vi "Balance.vi"() -> ()   [LabVIEW 2014]
uses:
  <userlib>/UCSD Robotics Lab/Robotics-Cape/LV/libroboticscape.lvlib
panel:
  in  "Fast Loop Gain Multiplier":dbl=1.0
  out "State":T1(ring)
  in  "Slow Loop Gain Multiplier":dbl=1.0
  in  "Gamma Setpoint":dbl
  in  "Phi Setpoint":dbl step=0.25
  in  "Steering On/off":bool=TRUE
  out "Slow Loop State":T2 {"Phi Setpoint" format="%#_13g"; "Phi" format="%#_4g"; "error Phi" format="%#_4g"; "Gamma" format="%#_4g"}
  out "Actual Loop rate (Hz)":dbl format="%#_4g"
  out "Armed Status":bool
  out "Fast Loop State":T3 {"Theta (Deg)" format="%#_3g"; "Theta (Rad)" format="%#_3g"; "eTheta" format="%#_3g"; "Steering U" format="%#_2g"}
  in  "Controller - User Input":T4={"Num Fast Loop"=[-5.391, 10.21, -4.829], "Den Fast Loop"=[1.0, -1.702, 0.702], "Fast Loop Gain"=1.0, "IMU_sample_rate"=200, "Num Slow Loop"=[0.28, -0.5581, 0.2781], "Den Slow Loop"=[1.0, -1.86, 0.8605], "Slow Loop Gain"=1.0, "Slow Loop sample rate"=100.0} {"Slow Loop sample rate" min=4.0 max=200.0; "IMU_sample_rate" min=4 max=200}
  in  "Steering PID Gains":T5={"proportional"=0.1, "integral"=0.05, "derivative"=0.0}
  out "Slow Loop Gains":T6
  out "Commanded  Slow Loop Sample rate":dbl
  in  "Controller Select":T7(ring)=enum."User Defined" caption="Enum"
  out "Fast Loop Gains":T8
  in  "Display Slow Loop":bool
  in  "Display Fast Loop":bool
  out "U Plot":cluster{"U saturated":sgl, "U":dbl}(graph)
  out "Theta Ref":cluster{"Filtered x":dbl, "val out":sgl}(graph)
  out "Slower Loop (Hz)":dbl format="%#_4g"
  out "Theta Plot":dbl(graph)
  out "IMU_sample_rate":i32=200
  in  "stop":bool
  # "Always stop the VI using the rectangular STOP button below, never with the round stopsign (Abort)"
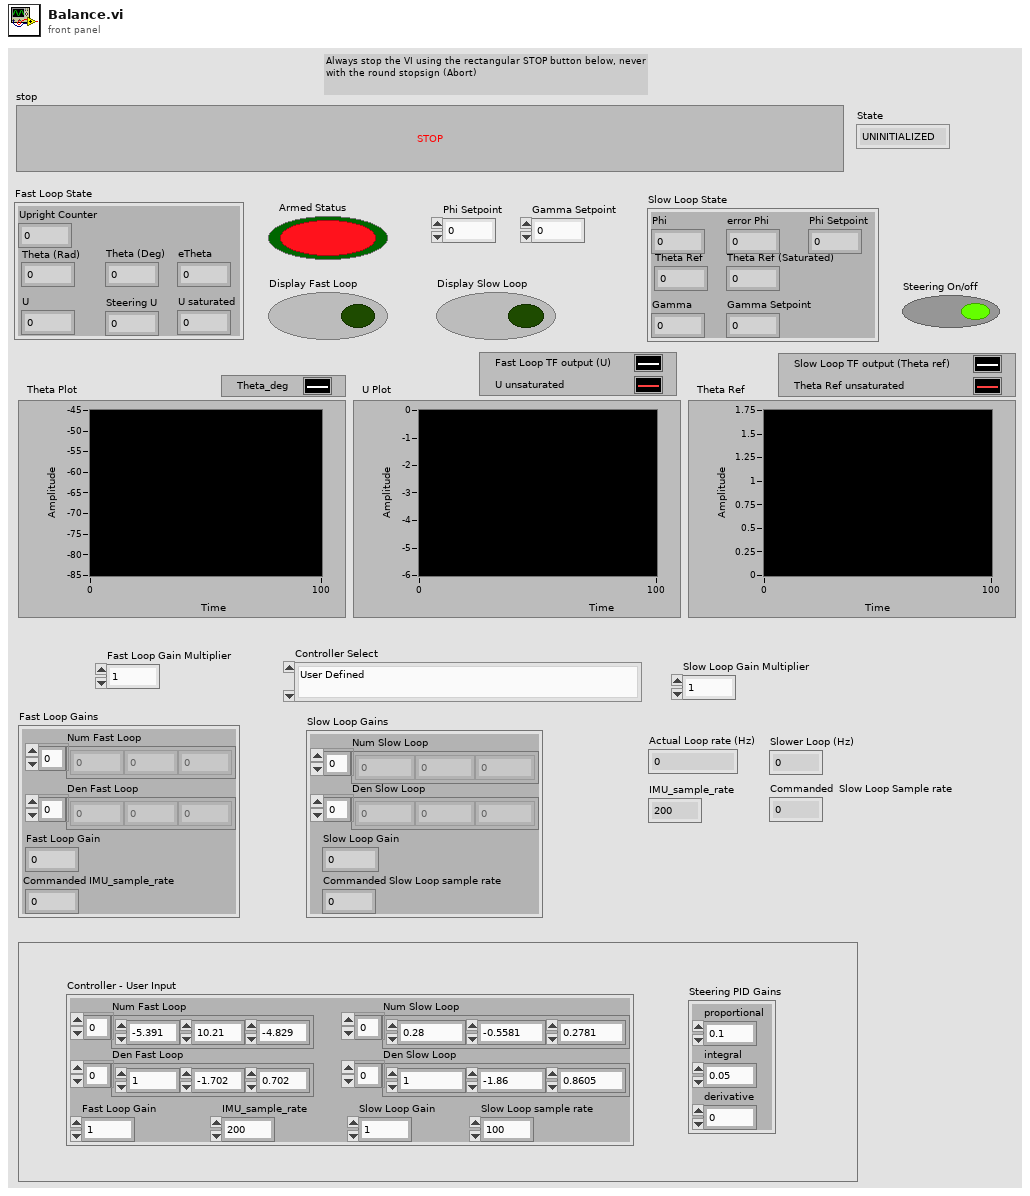
[diagram p1: front panel]
types:
  T1 = enum16{"UNINITIALIZED", "RUNNING", "PAUSED", "EXITING"}
  T2 = cluster{"Phi":dbl, "error Phi":dbl, "Gamma":dbl, "Theta Ref":dbl, "Theta Ref (Saturated)":sgl, "Gamma Setpoint":dbl, "Phi Setpoint":dbl}
  T3 = cluster{"Upright Counter":dbl, "Theta (Deg)":dbl, "Theta (Rad)":dbl, "eTheta":dbl, "U":dbl, "Steering U":dbl, "U saturated":sgl}
  T4 = cluster{"Num Fast Loop":dbl[], "Den Fast Loop":dbl[], "Fast Loop Gain":dbl, "IMU_sample_rate":i32, "Num Slow Loop":dbl[], "Den Slow Loop":dbl[], "Slow Loop Gain":dbl, "Slow Loop sample rate":dbl}
  T5 = cluster{"proportional":dbl, "integral":dbl, "derivative":dbl}
  T6 = cluster{"Num Slow Loop":dbl[], "Den Slow Loop":dbl[], "Slow Loop Gain":dbl, "Commanded Slow Loop sample rate":dbl}
  T7 = enum16{"100hz/50hz", "100hz/100hz", "200hz/200hz", "200hz/20hz", "User Defined"}
  T8 = cluster{"Num Fast Loop":dbl[], "Den Fast Loop":dbl[], "Fast Loop Gain":dbl, "Commanded IMU_sample_rate":i32}
  T9 = cluster{"accel[0]":sgl, "accel[1]":sgl, "accel[2]":sgl, "gyro[0]":sgl, "gyro[1]":sgl, "gyro[2]":sgl, "mag[0]":sgl, "mag[1]":sgl, "mag[2]":sgl, "temp":sgl, "raw_gyro[0]":i16, "raw_gyro[1]":i16, "raw_gyro[2]":i16, "raw_accel[0]":i16, "raw_accel[1]":i16, "raw_accel[2]":i16, "accel_to_ms2":sgl, "gyro_to_degs":sgl, "dmp_quat[0]":sgl, "dmp_quat[1]":sgl, "dmp_quat[2]":sgl, "dmp_quat[3]":sgl, "dmp_TaitBryan[0]":sgl, "dmp_TaitBryan[1]":sgl, "dmp_TaitBryan[2]":sgl, "fused_quat[0]":sgl, "fused_quat[1]":sgl, "fused_quat[2]":sgl, "fused_quat[3]":sgl, "fused_TaitBryan[0]":sgl, "fused_TaitBryan[1]":sgl, "fused_TaitBryan[2]":sgl, "compass_heading":sgl, "compass_heading_raw":sgl}
  T10 = enum16{"UNINITIALIZED", "RUNING", "PAUSED", "EXITING"}
  T11 = cluster{"Num Fast Loop":dbl[], "Den Fast Loop":dbl[], "Fast Loop Gain 3":dbl, "IMU_sample_rate":i32}
  T12 = cluster{"Upright Counter":dbl, "Theta (Deg)":dbl, "Theta (Rad)":dbl, "eTheta":dbl, "U":dbl, "Steering output":dbl, "U saturated":sgl}
  T13 = cluster{"Num Slow Loop":dbl[], "Den Slow Loop":dbl[], "Slow Loop Gain":dbl, "Commanded Slow Sample rate":dbl}
  T14 = cluster{"Theta Ref":dbl, "Theta Ref (Saturated)":sgl}
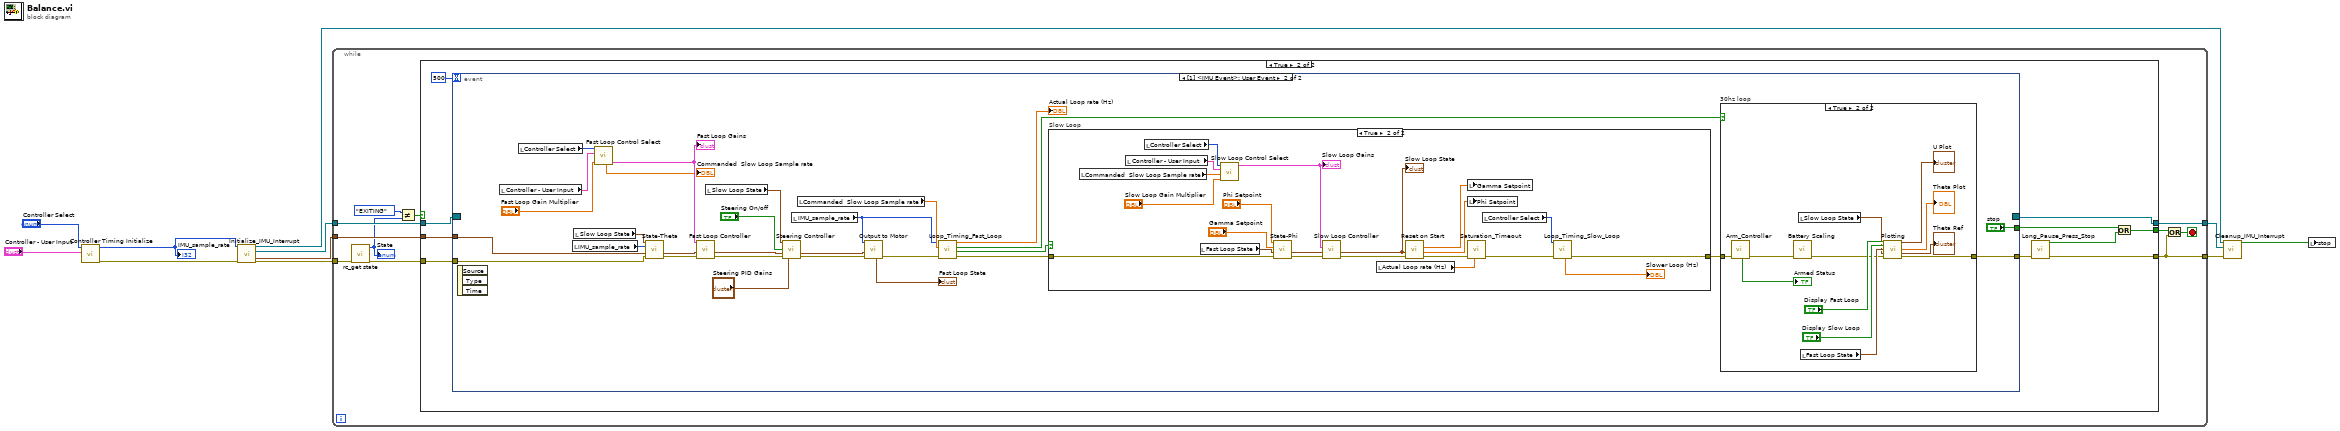
[diagram p0: block diagram]
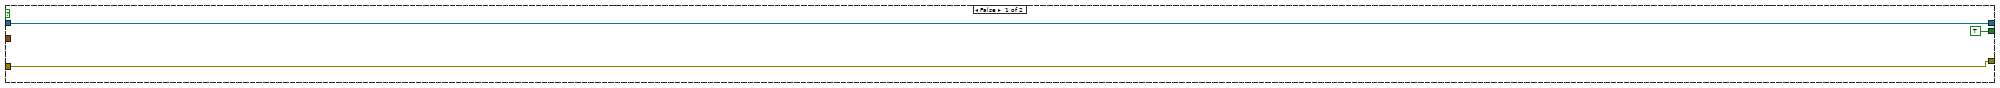
[diagram p2: hidden frame]
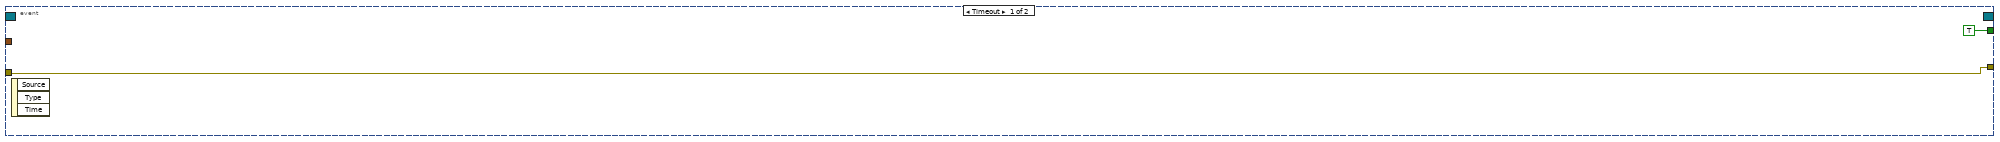
[diagram p3: hidden frame]
diagram:
  n1 = call "Controller Timing Initialize.vi"("Controller - User Input"="Controller - User Input", "Controller Select"="Controller Select") -> ("error out"=w2:errorcluster, "IMU_sample_rate"=w5:i32)  [unwired: 8 in]
  "IMU_sample_rate" <- w5
  n2 = call "Initialize_IMU_Interrupt.vi"("dmp_sample_rate"=w5, "error in (no error)"=w2) -> ("IMU Event"=w8:refnum<user-event>, "Event Registration Refnum"=w10:refnum<event-registration>, "IMU Data"=w6:T9, "error out"=w3:errorcluster)  [unwired: 10 in]
  n3 = while {
    tunnel: w3 -> [w17]
    tunnel: [w22] -> w7
    tunnel: [w20] -> w11
    tunnel: w10 -> [w21]
    tunnel: w6 -> [w18]
    stop <- w19 stop-if-true
    n4 = call <userlib>:"rc_get state.vi"("error in (no error)"=w17) -> ("error out"=w16:errorcluster, "function return"=w12:u32)  [unwired: 9 in]
    "State" <- w12
    n5 = Not Equal?(x=T10."EXITING" ("State 2"), y=w12) -> (x != y?=w14:bool)
    n6 = case shown="True" w14 {
      tunnel: [w24 w35] -> w22
      tunnel: w21 -> [w24 w33]
      tunnel: [w25 w29] -> w20
      tunnel: w18 -> [_ w32]
      tunnel: w16 -> [w25 w31]
      tunnel: [TRUE ("stop") w26] -> w13
      frame False {
      }
      frame True {
        n7 = event shown="[1] <IMU Event>: User Event" {
          selector: w33 -> [_ _]
          dyn-events: [_ _] -> w35
          timeout: 500 -> [_ _]
          tunnel: w31 -> [w37 w66]
          tunnel: [w37 w56] -> w30
          tunnel: w32 -> [_ w55]
          tunnel: [TRUE ("stop") "stop"] -> w27
          event Timeout {
            n8 = event-data() -> ()  [unwired: 1 in, 3 out]
          }
          event User Event {
            n9 = event-data() -> ()  [unwired: 1 in, 3 out]
            n10 = local read "Controller - User Input"() -> (w39:T4)
            n11 = local read "Controller Select"() -> (w43:T7)
            n12 = local read "IMU_sample_rate"() -> (w42:i32)
            n13 = local read "Slow Loop State"() -> (w45:T2)
            n14 = call "Fast Loop Control Select.vi"("Fast Loop Gain Multiplier"="Fast Loop Gain Multiplier", "Controller - User Input"=w39, "Controller Select"=w43) -> ("Fast Loop Controller"=w48:T11, "Slow Loop sample rate out"=→"Commanded  Slow Loop Sample rate":dbl)  [unwired: 7 in]
            "Fast Loop Gains" <- w48
            n15 = call "State-Theta.vi"("Slow Loop State in"=w45, "IMU_sample_rate"=w42, "IMU Data Struct in"=w55, "error in"=w66) -> ("Fast Loop State out"=w54:T12, "error out"=w65:errorcluster)  [unwired: 10 in]
            n16 = call "Fast Loop Controller.vi"("error in"=w65, "Fast Loop State in"=w54, "Fast Loop Controller in"=w48) -> ("error out"=w62:errorcluster, "Fast Loop State out"=w53:T12)  [unwired: 7 in]
            n17 = local read "Slow Loop State"() -> (w46:T2)
            n18 = call "Steering Controller.vi"("Slow Loop State in"=w46, "Steering On/off"="Steering On/off", "Fast Loop State in"=w53, "error in"=w62, "PID Gains in"="Steering PID Gains") -> ("Fast Loop State out"=w52:T12, "error out"=w61:errorcluster)  [unwired: 9 in]
            n19 = local read "IMU_sample_rate"() -> (w41:i32)
            n20 = local read "Commanded  Slow Loop Sample rate"() -> (w50:dbl)
            n21 = call "Output to Motor.vi"("error in (no error)"=w61, "Fast Loop State in"=w52, "IMU_sample_rate"=w41) -> ("error out"=w64:errorcluster, "Fast Loop State out"=→"Fast Loop State":T12)  [unwired: 7 in]
            n22 = call "Loop_Timing_Fast_Loop.vi"("error in"=w64, "Slow Loop sample rate in"=w50, "IMU_sample_rate in"=w41) -> ("error out"=w58:errorcluster, "Slow Loop Start"=w63:bool, "30hz Start"=w60:bool, "Hz"=→"Actual Loop rate (Hz)":dbl)  [unwired: 5 in]
            n23 = case "Slow Loop" shown="True" w63 {
              tunnel: [w80 w101] -> w57
              tunnel: w58 -> [w80 w96]
              frame False {
              }
              frame True {
                n24 = local read "Commanded  Slow Loop Sample rate"() -> (w99:dbl)
                n25 = local read "Controller - User Input"() -> (w98:T4)
                n26 = local read "Controller Select"() -> (w81:T7)
                n27 = local read "Fast Loop State"() -> (w97:T3)
                n28 = call "Slow Loop Control Select.vi"("Slow Loop Gain Multiplier"="Slow Loop Gain Multiplier", "Commanded Slow Sample rate"=w99, "Controller - User Input"=w98, "Controller Select"=w81) -> ("Slow Loop Gains"=w86:T13)  [unwired: 7 in]
                "Slow Loop Gains" <- w86
                n29 = call "State-Phi.vi"("error in (no error)"=w96, "Fast Loop State in"=w97, "Gamma Setpoint"="Gamma Setpoint", "Phi Setpoint"="Phi Setpoint") -> ("error out"=w100:errorcluster, "Slow Loop State out"=w85:T2)  [unwired: 6 in]
                n30 = call "Slow Loop Controller.vi"("error in"=w100, "Slow Loop State in"=w85, "Slow Loop Gains"=w86) -> ("error out"=w94:errorcluster, "Slow Loop State out"=w87:T2)  [unwired: 5 in]
                "Slow Loop State" <- w87
                n31 = local read "Actual Loop rate (Hz)"() -> (w95:dbl)
                n32 = call "Reset on Start.vi"("error in (no error)"=w94, "Slow Loop State"=w87) -> ("error out"=w93:errorcluster, "Phi Setpoint"=w89:dbl, "Gamma Setpoint"=w90:dbl)  [unwired: 6 in, 1 out]
                n33 = local write "Gamma Setpoint"(w90) -> ()
                n34 = local write "Phi Setpoint"(w89) -> ()
                n35 = call "Saturation_Timeout.vi"("Hz"=w95, "error in"=w93) -> ("error out"=w92:errorcluster)  [unwired: 9 in]
                n36 = local read "Controller Select"() -> (w82:T7)
                n37 = call "Loop_Timing_Slow_Loop.vi"("error in"=w92, "Controller Select"=w82) -> ("error out"=w101:errorcluster, "Hz"=→"Slower Loop (Hz)":dbl)  [unwired: 6 in, 2 out]
              }
            }
            n38 = case "30hz loop" shown="True" w60 {
              tunnel: w57 -> [w67 w79]
              tunnel: [w67 w78] -> w56
              frame False {
              }
              frame True {
                n39 = call "Arm_Controller.vi"("error in (no error)"=w79) -> ("error out"=w70:errorcluster, "Arm Controller"=→"Armed Status":bool)  [unwired: 8 in, 1 out]
                n40 = call "Battery Scaling.vi"("error in (no error)"=w70) -> ("error out"=w69:errorcluster)  [unwired: 9 in, 1 out]
                n41 = local read "Slow Loop State"() -> (w68:T2)
                n42 = local read "Fast Loop State"() -> (w75:T3)
                n43 = call "Plotting.vi"("Display Fast Loop"="Display Fast Loop", "Display Slow Loop"="Display Slow Loop", "Fast Loop State in"=w75, "Slow Loop State in"=w68, "error in (no error)"=w69) -> ("U plot"=→"U Plot":cluster{"U saturated":sgl, "U":dbl}, "Theta (Deg)"=→"Theta Plot":dbl, "Theta Ref Plot"=→"Theta Ref":T14, "error out"=w78:errorcluster)  [unwired: 7 in]
              }
            }
          }
        }
        n44 = call "Long_Pause_Press_Stop.vi"("error in (no error)"=w30) -> ("error out"=w29:errorcluster, "Stop"=w28:bool)  [unwired: 9 in]
        n45 = Or(x=w27, y=w28) -> (x .or. y?=w26:bool)
      }
    }
    n46 = Or(x=w13, y=w20) -> (x .or. y?=w19:bool)
  }
  n47 = call "Cleanup_IMU_Interrupt.vi"("error in (no error)"=w11, "Event Registration Refnum 2"=w7, "IMU Event"=w8) -> ("Stop Local Variabl"=w9:bool)  [unwired: 6 in]
  n48 = local write "stop"(w9) -> ()
